vi "Main Vending Machine.vi"() -> ()   [LabVIEW 2017]
uses:
  Controls/Pick up.ctl
  Controls/Refrescos.ctl
  Controls/Coins.ctl
  Controls/Control.ctl
  Controls/Data.ctl
  Controls/Data_In.ctl
  Controls/Venta.ctl
panel:
  in  "Help":bool
  out "Status":string
  in  "Coins":T1
  in  "Items":T2
  in  "Change/Pick Up":bool
  out "Pick up":T3
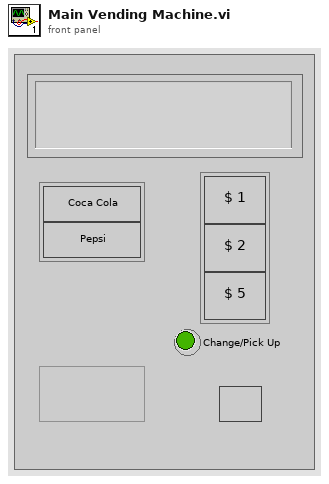
[diagram p1: front panel]
types:
  T1 = typedef "Coins.ctl" = cluster{"1 coin":bool, "2 coins":bool, "5 coins":bool}
  T2 = typedef "Refrescos.ctl" = cluster{"Coca":bool, "Pepsi":bool}
  T3 = typedef "Pick up.ctl" = bool
  T4 = typedef "Control.ctl" = enum16{"Inicializar", "Event Handler", "Sumar", "Producto", "Change/Pick Up", "Help", "Stop"}
  T5 = typedef "Data_In.ctl" = cluster{"Grand Total":i32, "Coca Cola":i32, "Pepsi":i32, "M5":i32, "M2":i32, "M1":i32}
  T6 = typedef "Data.ctl" = enum16{"Grand Total", "Coca-Cola", "Pepsi", "M1", "M2", "M5"}
  T7 = typedef "Venta.ctl" = enum16{"V_coca", "V_pepsi"}
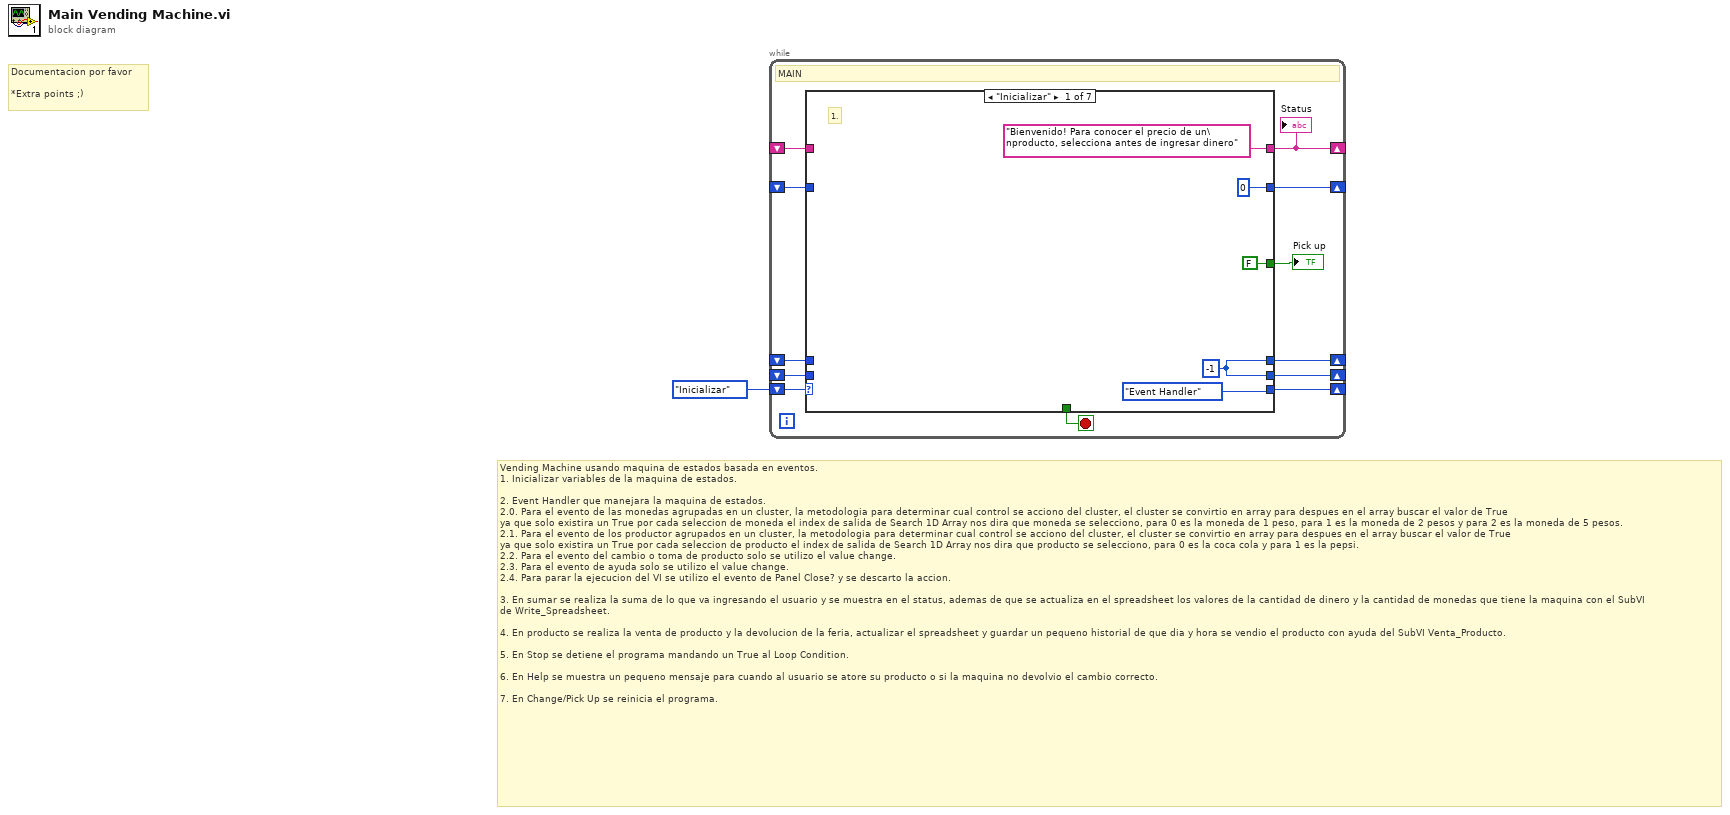
[diagram p0: block diagram]
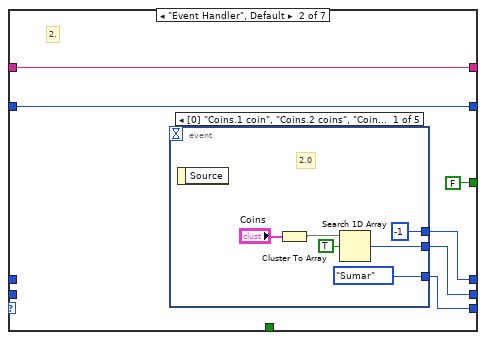
[diagram p2: hidden frame]
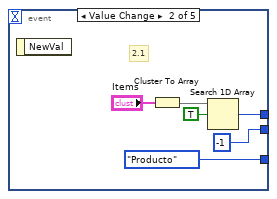
[diagram p3: hidden frame]
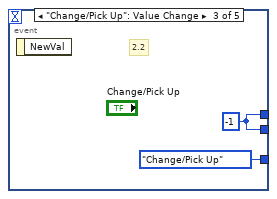
[diagram p4: hidden frame]
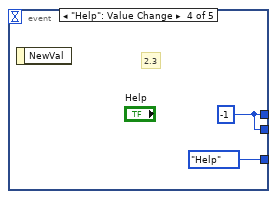
[diagram p5: hidden frame]
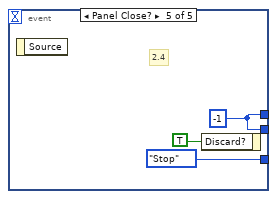
[diagram p6: hidden frame]
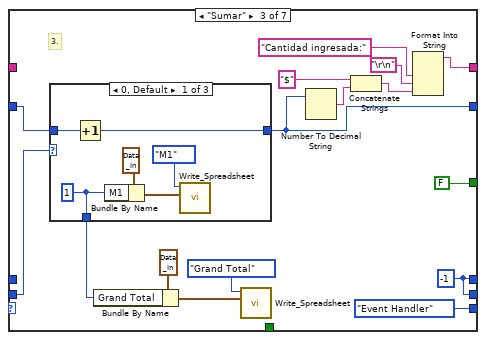
[diagram p7: hidden frame]
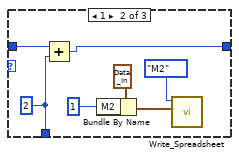
[diagram p8: hidden frame]
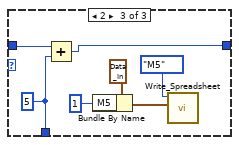
[diagram p9: hidden frame]
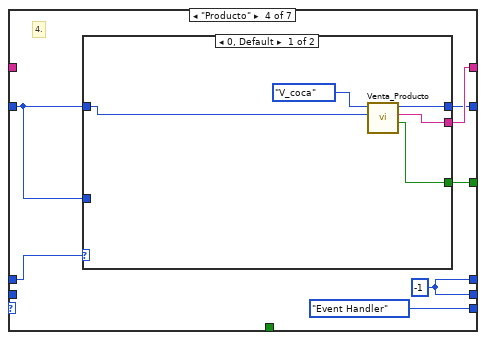
[diagram p10: hidden frame]
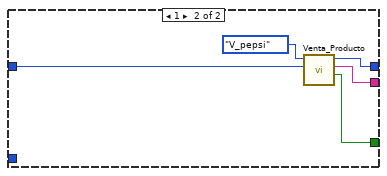
[diagram p11: hidden frame]
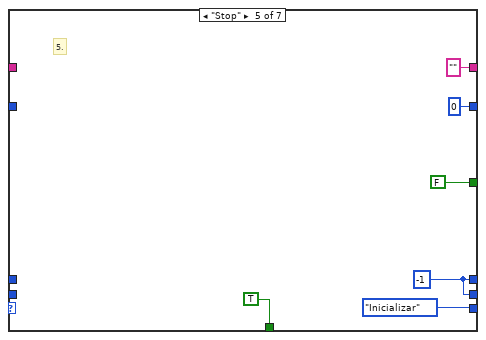
[diagram p12: hidden frame]
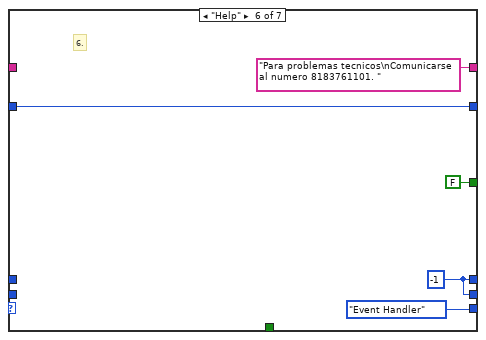
[diagram p13: hidden frame]
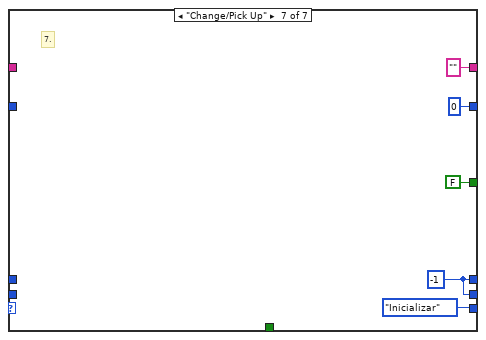
[diagram p14: hidden frame]
diagram:
  # "Vending Machine usando maquina de estados basada en eventos.\n1. Inicializar variables de la maquina de estados.\n\n2. Event Handler que manejara la maquina de estados.\n2.0. Para el evento de las monedas agrupadas en un cluster, la metodologia para determinar cual control se acciono del cluster, el cluster se convirtio en array para despues en el array buscar el valor de True\nya que solo existira un True por cada seleccion de moneda el index de salida de Search 1D Array nos dira que moneda se selecciono, para 0 es la moneda de 1 peso, para 1 es la moneda de 2 pesos y para 2 es la moneda de 5 pesos.\n2.1. Para el evento de los productor agrupados en un cluster, la metodologia para determinar cual control se acciono del cluster, el cluster se convirtio en array para despues en el array buscar el valor de True\nya que solo existira un True por cada seleccion de producto el index de salida de Search 1D Array nos dira que producto se selecciono, para 0 es la coca cola y para 1 es la pepsi.\n2.2. Para el evento del cambio o toma de producto solo se utilizo el value change.\n2.3. Para el evento de ayuda solo se utilizo el value change.\n2.4. Para parar la ejecucion del VI se utilizo el evento de Panel Close? y se descarto la accion.\n\n3. En sumar se realiza la suma de lo que va ingresando el usuario y se muestra en el status, ademas de que se actualiza en el spreadsheet los valores de la cantidad de dinero y la cantidad de monedas que tiene la maquina con el SubVI\nde Write_Spreadsheet. \n\n4. En producto se realiza la venta de producto y la devolucion de la feria, actualizar el spreadsheet y guardar un pequeno historial de que dia y hora se vendio el producto con ayuda del SubVI Venta_Producto.\n\n5. En Stop se detiene el programa mandando un True al Loop Condition.\n\n6. En Help se muestra un pequeno mensaje para cuando al usuario se atore su producto o si la maquina no devolvio el cambio correcto.\n\n7. En Change/Pick Up se reinicia el programa."
  # "Documentacion por favor\n\n*Extra points ;)"
  n1 = while {
    shift-right: [w12] -> _
    shift-left: Control."Inicializar" -> [w13]
    shift-right: [w10] -> _
    shift-left: _ -> [w9]
    shift-right: [w3] -> _
    shift-left: _ -> [w8]
    shift-right: [w7] -> _
    shift-left: _ -> [w6]
    shift-right: [w5] -> _
    shift-left: _ -> [w4]
    stop <- w11 stop-if-true
    # "MAIN"
    n2 = case shown="\"Inicializar\"" w13 {
      tunnel: [Control."Event Handler" w24 Control."Event Handler" Control."Event Handler" Control."Inicializar" Control."Event Handler" Control."Inicializar"] -> w12
      tunnel: [_ _ _ _ TRUE ("Discard?") _ _] -> w11
      tunnel: [w15 w23 w49 w83 w100 w106 w109] -> w10
      tunnel: w9 -> [_ _ w59 _ _ _ _]
      tunnel: [0 w22 w50 w81 0 ("Feria") w104 0 ("Feria")] -> w3
      tunnel: w8 -> [_ w22 w58 w82 _ w104 _]
      tunnel: ["Bienvenido! Para conocer el precio de un\nproducto, selecciona antes de ingresar dinero" ("Line 1") w19 w47 w84 "" ("Mensaje") "Para problemas tecnicos\nComunicarse al numero 8183761101. " ("Mensaje") "" ("Mensaje")] -> w7
      tunnel: w6 -> [_ w19 _ _ _ _ _]
      tunnel: [w15 w21 w49 w83 w100 w106 w109] -> w5
      tunnel: w4 -> [_ _ _ w85 _ _ _]
      tunnel: [FALSE ("Discard?") FALSE ("Discard?") FALSE ("Discard?") w80 FALSE ("Discard?") FALSE ("Discard?") FALSE ("Discard?")] -> w2
      frame "Inicializar" {
        w15 = -1 ("index of element")
        # "1."
      }
      frame "Event Handler", Default {
        # "2."
        n3 = event shown="[0] \"Coins.1 coin\", \"Coins.2 coins\", \"Coins.5 coins\": Value Change" {
          selector: _ -> [_ _ _ _ _]
          dyn-events: _ -> [_ _ _ _ _]
          timeout: _ -> [_ _ _ _ _]
          tunnel: [Control."Sumar" Control."Producto" Control."Change/Pick Up" Control."Help" Control."Stop"] -> w24
          tunnel: [w29 -1 ("index of element") w37 w40 w42] -> w23
          tunnel: [-1 ("index of element") w33 w37 w40 w42] -> w21
          event Value Change {
            # "2.0"
            n4 = event-data() -> ()  [unwired: 1 in, 1 out]
            n5 = Cluster To Array(cluster="Coins") -> (array=w27:bool[])
            n6 = Search 1D Array(1D array=w27, element=TRUE) -> (index of element=w29:i32)  [unwired: 1 in]
          }
          event Value Change {
            # "2.1"
            n7 = event-data() -> ()  [unwired: 1 in, 1 out]
            n8 = Cluster To Array(cluster="Items") -> (array=w35:bool[])
            n9 = Search 1D Array(1D array=w35, element=TRUE) -> (index of element=w33:i32)  [unwired: 1 in]
          }
          event "Change/Pick Up": Value Change {
            w37 = -1 ("index of element")
            # "2.2"
            n10 = event-data() -> ()  [unwired: 1 in, 1 out]
          }
          event "Help": Value Change {
            w40 = -1 ("index of element")
            # "2.3"
            n11 = event-data() -> ()  [unwired: 1 in, 1 out]
          }
          event Panel Close? {
            w42 = -1 ("index of element")
            # "2.4"
            n12 = event-data() -> ()  [unwired: 1 in, 1 out]
            n13 = event-data("Discard?"=TRUE) -> ()  [unwired: 1 in, 1 out]
          }
        }
      }
      frame "Sumar" {
        w49 = -1 ("y")
        # "3."
        n14 = case shown="0, Default" w59 {
          tunnel: [w64 w72 w78] -> w50
          tunnel: w58 -> [w65 w71 w79]
          tunnel: [w63 w70 w77] -> w53
          frame 0, Default {
            w63 = 1 ("y")
            n15 = Increment(x=w65) -> (x+1=w64:i32)
            n16 = Bundle By Name(cluster=T5 {"Grand Total"=0, "Coca Cola"=0, "Pepsi"=0, "M5"=0, "M2"=0, "M1"=0} ("Data In"), "M1"=w63) -> (w61:T5)
            n17 = call "Write_Spreadsheet.vi"("Data In"=w61, "Data"=Data."M1" ("Enum")) -> ()  [unwired: 10 in]
          }
          frame 1 {
            w70 = 2 ("y")
            n18 = Add(x=w71, y=w70) -> (x+y=w72:i32)
            n19 = Bundle By Name(cluster=T5 {"Grand Total"=0, "Coca Cola"=0, "Pepsi"=0, "M5"=0, "M2"=0, "M1"=0} ("Data In"), "M2"=1 ("y")) -> (w68:T5)
            n20 = call "Write_Spreadsheet.vi"("Data In"=w68, "Data"=Data."M2" ("Enum")) -> ()  [unwired: 10 in]
          }
          frame 2 {
            w77 = 5 ("y")
            n21 = Add(x=w79, y=w77) -> (x+y=w78:i32)
            n22 = Bundle By Name(cluster=T5 {"Grand Total"=0, "Coca Cola"=0, "Pepsi"=0, "M5"=0, "M2"=0, "M1"=0} ("Data In"), "M5"=1 ("y")) -> (w76:T5)
            n23 = call "Write_Spreadsheet.vi"("Data In"=w76, "Data"=Data."M5" ("Enum")) -> ()  [unwired: 10 in]
          }
        }
        n24 = Bundle By Name(cluster=T5 {"Grand Total"=0, "Coca Cola"=0, "Pepsi"=0, "M5"=0, "M2"=0, "M1"=0} ("Data In"), "Grand Total"=w53) -> (w55:T5)
        n25 = call "Write_Spreadsheet.vi"("Data In"=w55, "Data"=Data."Grand Total" ("Enum")) -> ()  [unwired: 10 in]
        n26 = Number To Decimal String(number=w50) -> (decimal integer string=w51:string)  [unwired: 1 in]
        n27 = Concatenate Strings("$" ("string"), w51) -> (w45:string)
        n28 = Format Into String("Cantidad ingresada:" ("Line 1"), "\r\n", w45) -> (resulting string=w47:string)  [unwired: 3 in, 1 out]
      }
      frame "Producto" {
        w83 = -1 ("y")
        # "4."
        n29 = case shown="0, Default" w85 {
          tunnel: w82 -> [_ _]
          tunnel: [w88 w92] -> w84
          tunnel: w82 -> [w91 w96]
          tunnel: [w89 w94] -> w81
          tunnel: [w87 w93] -> w80
          frame 0, Default {
            n30 = call "Venta_Producto.vi"("Ingresado"=w91, "Venta"=Venta."V_coca") -> ("Product?"=w87:bool, "Mensaje"=w88:string, "Feria"=w89:i32)  [unwired: 7 in]
          }
          frame 1 {
            n31 = call "Venta_Producto.vi"("Ingresado"=w96, "Venta"=Venta."V_pepsi") -> ("Product?"=w93:bool, "Mensaje"=w92:string, "Feria"=w94:i32)  [unwired: 7 in]
          }
        }
      }
      frame "Stop" {
        w100 = -1 ("y")
        # "5."
      }
      frame "Help" {
        w106 = -1 ("y")
        # "6."
      }
      frame "Change/Pick Up" {
        w109 = -1 ("y")
        # "7."
      }
    }
    "Status" <- w7
    "Pick up" <- w2
  }
